vi "VIP_Post-Uninstall Custom Action.vi"(10 "Variant":variant) -> (0 "error out":errorcluster)   [LabVIEW 2021]
uses:
  <vilib>/zip/NI_Unzip.lvlib
  <vilib>/Utility/config.llb/NI_LVConfig.lvlib
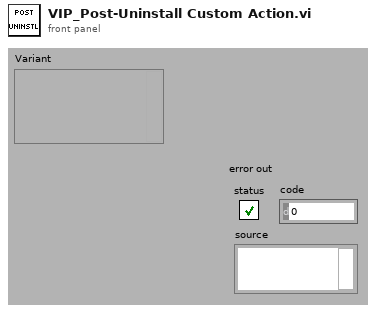
[diagram p1: front panel]
types:
  T1 = typedef "NI_LVConfig.lvlib/Config Data RefNum.ctl" = refnum<k1>
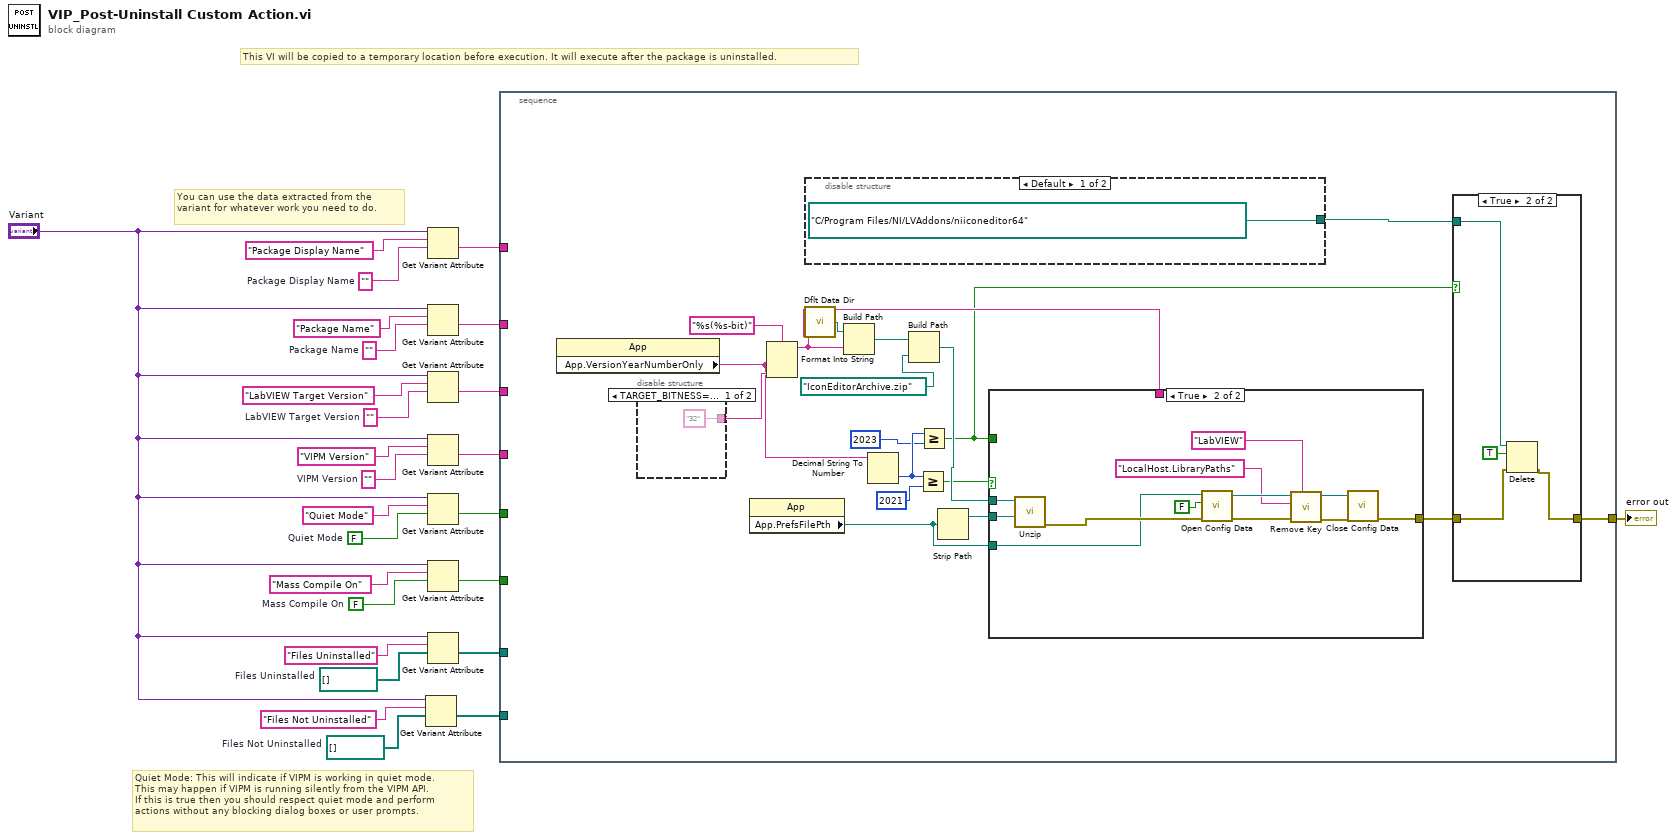
[diagram p0: block diagram]
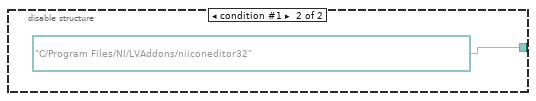
[diagram p2: hidden frame]
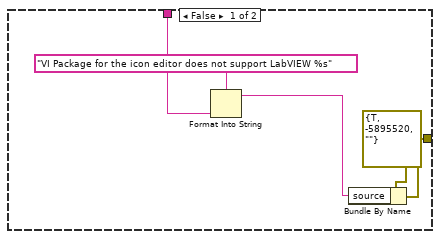
[diagram p4: hidden frame]
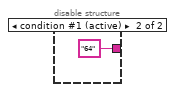
[diagram p5: hidden frame]
diagram:
  w2 = path[] []  # Files Not Uninstalled
  w3 = path[] []  # Files Uninstalled
  w9 = FALSE  # Mass Compile On
  w10 = ""  # Package Display Name
  w17 = FALSE  # Quiet Mode
  w20 = ""  # VIPM Version
  w22 = ""  # LabVIEW Target Version
  w24 = ""  # Package Name
  # "You can use the data extracted from the variant for whatever work you need to do."
  # "Quiet Mode: This will indicate if VIPM is working in quiet mode.\nThis may happen if VIPM is running silently from the VIPM API.\nIf this is true then you should respect quiet mode and perform\nactions without any blocking dialog boxes or user prompts."
  # "This VI will be copied to a temporary location before execution. It will execute after the package is uninstalled."
  n1 = Get Variant Attribute(Variant="Variant", name="Files Not Uninstalled", default value (empty Variant)=w2) -> (value=w7:path[])  [unwired: 1 in, 3 out]
  n2 = Get Variant Attribute(Variant="Variant", name="Package Display Name", default value (empty Variant)=w10) -> (value=w16:string)  [unwired: 1 in, 3 out]
  n3 = Get Variant Attribute(Variant="Variant", name="Package Name", default value (empty Variant)=w24) -> (value=w15:string)  [unwired: 1 in, 3 out]
  n4 = Get Variant Attribute(Variant="Variant", name="LabVIEW Target Version", default value (empty Variant)=w22) -> (value=w14:string)  [unwired: 1 in, 3 out]
  n5 = Get Variant Attribute(Variant="Variant", name="VIPM Version", default value (empty Variant)=w20) -> (value=w13:string)  [unwired: 1 in, 3 out]
  n6 = Get Variant Attribute(Variant="Variant", name="Quiet Mode", default value (empty Variant)=w17) -> (value=w12:bool)  [unwired: 1 in, 3 out]
  n7 = Get Variant Attribute(Variant="Variant", name="Mass Compile On", default value (empty Variant)=w9) -> (value=w11:bool)  [unwired: 1 in, 3 out]
  n8 = Get Variant Attribute(Variant="Variant", name="Files Uninstalled", default value (empty Variant)=w3) -> (value=w6:path[])  [unwired: 1 in, 3 out]
  n9 = stacked-sequence {
    tunnel: w16 -> [_]
    tunnel: w15 -> [_]
    tunnel: w14 -> [_]
    tunnel: w13 -> [_]
    tunnel: w12 -> [_]
    tunnel: w11 -> [_]
    tunnel: w6 -> [_]
    tunnel: w7 -> [_]
    tunnel: [w30] -> w1
    frame #0 {
      n10 = property class="App"() -> ("App.VersionYearNumberOnly"=w29:string)  [unwired: 2 in, 2 out]
      n11 = disable-structure shown="TARGET_BITNESS==32" {
        disable-tunnel: ["32" "64"] -> w39
        frame condition #0 {
        }
        frame condition #1 (active) {
        }
      }
      n12 = property class="App"() -> ("App.PrefsFilePth"=w37:path)  [unwired: 2 in, 2 out]
      n13 = Format Into String(format string="%s(%s-bit)", w29, w39) -> (resulting string=w32:string)  [unwired: 2 in, 1 out]
      n14 = call <vilib>:"Dflt Data Dir.vi"() -> ("App:Default Data Directory"=w43:path)
      n15 = disable-structure shown="Default" {
        disable-tunnel: [path "C:/Program Files/NI/LVAddons/niiconeditor64" ("Destination[i] Paths (Absolute)") path "C:/Program Files/NI/LVAddons/niiconeditor32" ("Destination[i] Paths (Absolute)")] -> w27
        frame condition #0 (active) {
        }
        frame condition #1 {
        }
      }
      n16 = Build Path(base path=w43, name or relative path=w32) -> (appended path=w42:path)
      n17 = Decimal String To Number(string=w29) -> (number=w34:i32)  [unwired: 2 in, 1 out]
      n18 = Build Path(base path=w42, name or relative path=path "IconEditorArchive.zip") -> (appended path=w40:path)
      n19 = Greater Or Equal?(x=w34, y=2021) -> (x >= y?=w35:bool)
      n20 = Greater Or Equal?(x=w34, y=2023) -> (x >= y?=w28:bool)
      n21 = Strip Path(path=w37) -> (stripped path=w38:path)  [unwired: 1 out]
      n22 = case shown="True" w35 {
        tunnel: w40 -> [_ w68]
        tunnel: [w53 w67] -> w31
        tunnel: w38 -> [_ w66]
        tunnel: w37 -> [_ w64]
        tunnel: w28 -> [_ _]
        tunnel: w32 -> [w56 _]
        frame False {
          n23 = Format Into String(format string="VI Package for the icon editor does not support LabVIEW %s", w56) -> (resulting string=w52:string)  [unwired: 2 in, 1 out]
          n24 = Bundle By Name(cluster=errorcluster {"status"=TRUE, "code"=-5895520, "source"=""} ("error out"), "source"=w52) -> (w53:errorcluster)
        }
        frame True {
          n25 = call <vilib>:"Unzip.vi"("Target directory (same as Zip file if empty)"=w66, "Zip file"=w68) -> ("error out"=w65:errorcluster)  [unwired: 7 in, 2 out]
          n26 = call <vilib>:"Open Config Data.vi"("error in (no error)"=w65, "create file if necessary (T)"=FALSE, "configuration file path"=w64) -> ("error out"=w63:errorcluster, "refnum"=w62:T1)  [unwired: 6 in, 1 out]
          n27 = call <vilib>:"Remove Key.vi"("section"="LabVIEW", "error in (no error)"=w63, "key"="LocalHost.LibraryPaths", "refnum"=w62) -> ("error out"=w59:errorcluster, "refnum out"=w58:T1)  [unwired: 5 in, 1 out]
          n28 = call <vilib>:"Close Config Data.vi"("error in (no error)"=w59, "refnum"=w58) -> ("error out"=w67:errorcluster)  [unwired: 8 in, 1 out]
        }
      }
      n29 = case shown="True" w28 {
        tunnel: w31 -> [w47 w51]
        tunnel: [w47 w50] -> w30
        tunnel: w27 -> [_ w48]
        frame False {
        }
        frame True {
          n30 = Delete(path (use dialog)=w48, entire hierarchy (F)=TRUE, error in=w51) -> (error out=w50:errorcluster)  [unwired: 2 in, 2 out]
        }
      }
    }
  }
  "error out" <- w1
